vi "ParseSCPI.vi"(11 "Input String":string=":CH1:SCAL 1.000000;:CH1:OFFS 0.000000;:CH1:COUP DC;:SEL:CH1 ON;") -> (2 "Data Out":string[](array[string]), 3 "Commands Out":string[](array[string]))   [LabVIEW 2020]
uses:
  <vilib>/Utility/error.llb/Trim Whitespace One-Sided.vi
panel:
  out "Full Commands":string[](array[string])
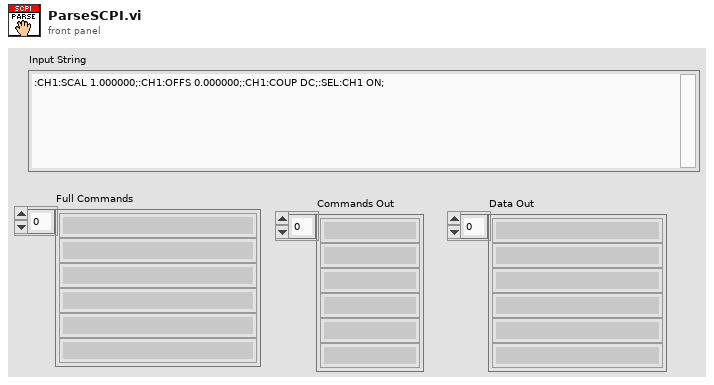
[diagram p1: front panel]
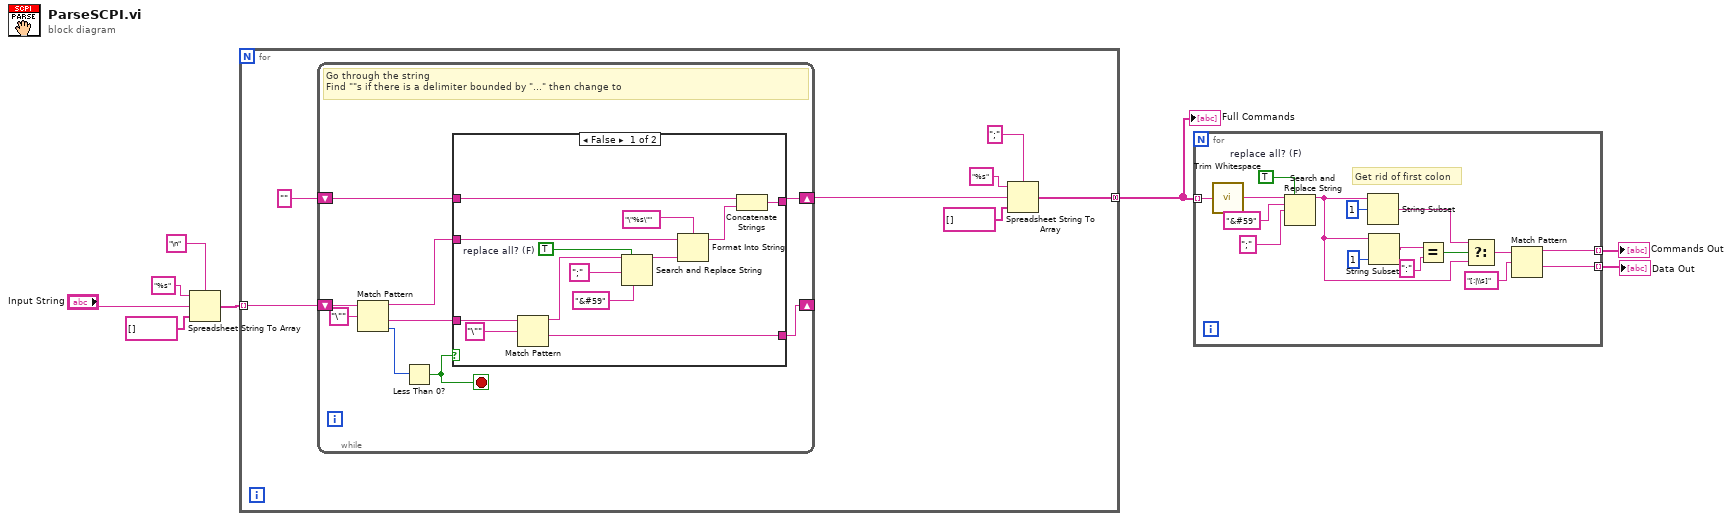
[diagram p0: block diagram]
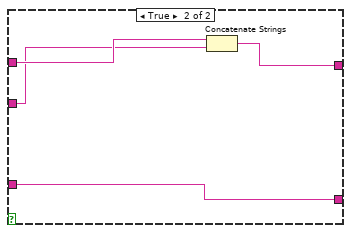
[diagram p2: hidden frame]
diagram:
  n1 = Spreadsheet String To Array(delimiter (Tab)="\n", format string="%s", spreadsheet string="Input String", array type (2D Dbl)=string[] []) -> (array=w1:string[])
  n2 = for {
    tunnel: w1 -> [w15] mode=indexing
    tunnel: [w9] -> w6 mode=concatenating
    n3 = while {
      shift-right: [w17] -> _
      shift-left: w15 -> [w23]
      shift-right: [w19] -> w10
      shift-left: "" -> [w18]
      stop <- w16 stop-if-true
      # "Go through the string\nFind \"\"s if there is a delimiter bounded by \"...\" then change to"
      n4 = Match Pattern(string=w23, regular expression="\"") -> (before substring=w20:string, after substring=w21:string, offset past match=w22:i32)  [unwired: 1 in, 1 out]
      n5 = Less Than 0?(x=w22) -> (x < 0?=w16:bool)
      n6 = case shown="False" w16 {
        tunnel: w21 -> [w36 w41]
        tunnel: w20 -> [w30 w38]
        tunnel: [w28 w39] -> w19
        tunnel: w18 -> [w27 w40]
        tunnel: [w26 w41] -> w17
        frame False {
          w35 = TRUE  # replace all? (F)
          n7 = Match Pattern(string=w36, regular expression="\"") -> (before substring=w32:string, after substring=w26:string)  [unwired: 1 in, 2 out]
          n8 = Search and Replace String(replace all?=w35, input string=w32, search string=";", replace string="&#59" ("replace string (\"\")")) -> (result string=w25:string)  [unwired: 4 in, 3 out]
          n9 = Format Into String(format string="\"%s\"", initial string=w30, w25) -> (resulting string=w29:string)  [unwired: 1 in, 1 out]
          n10 = Concatenate Strings(w27, w29) -> (w28:string)
        }
        frame True {
          n11 = Concatenate Strings(w40, w38) -> (w39:string)
        }
      }
    }
    n12 = Spreadsheet String To Array(delimiter (Tab)=";", format string="%s", spreadsheet string=w10, array type (2D Dbl)=string[] []) -> (array=w9:string[])
  }
  "Full Commands" <- w6
  n13 = for {
    tunnel: w6 -> [w57] mode=indexing
    tunnel: [w50] -> w8 mode=indexing
    tunnel: [w48] -> w7 mode=indexing
    w47 = TRUE  # replace all? (F)
    # "Get rid of first colon"
    n14 = call <vilib>:"Trim Whitespace.vi"("string"=w57) -> ("trimmed string"=w46:string)  [unwired: 1 in]
    n15 = Search and Replace String(replace all?=w47, input string=w46, search string="&#59" ("replace string (\"\")"), replace string=";" ("search string")) -> (result string=w45:string)  [unwired: 4 in, 3 out]
    n16 = String Subset(string=w45, offset (0)=1) -> (substring=w53:string)  [unwired: 1 in]
    n17 = String Subset(string=w45, length (rest)=1 ("length (rest)")) -> (substring=w42:string)  [unwired: 1 in]
    n18 = Equal?(x=w42, y=":" ("delimiter (Tab)")) -> (x = y?=w54:bool)
    n19 = Select(t=w53, s=w54, f=w45) -> (s? t:f=w51:string)
    n20 = Match Pattern(string=w51, regular expression="[:|\\s]") -> (before substring=w50:string, after substring=w48:string)  [unwired: 1 in, 2 out]
  }
  "Commands Out" <- w8
  "Data Out" <- w7
